vi "ContourExtraction.vi"() -> ()   [LabVIEW 2014]
doc: "This example shows how to use the Edge Tool in NI Vision. The Edge Tool finds edges (or sharp transitions in the pixels values) along a given line or ROI profile. The Edge Tool is a precursor function to many of the gauging and inspection tasks. For example, the location of the edges found along a line profile across an object can interpreted as the boundaries of the object whose dimensions have to be measured for a gauging application or the presence of a crack in the surface of an object for an inspection application."
uses:
  <vilib>/vision/Contour.llb/IMAQ Contour Curve Extraction.ctl
  <vilib>/vision/Contour.llb/IMAQ Connect Range Setting.ctl
  <vilib>/vision/NI_Vision_Development_Module.lvlib
panel:
  in  "Contour Selection":T1(ring)
  in  "Search Direction":T2(ring)
  in  "Curve Connection":T3[](array[typedef])=[{"Match Constraints"=0, "Min"=0.0, "Max"=25.0}, {"Match Constraints"=1, "Min"=0.0, "Max"=180.0}, {"Match Constraints"=2, "Min"=0.0, "Max"=25.0}, {"Match Constraints"=3, "Min"=0.0, "Max"=180.0}] {"Max" format="%.2f"; "Min" format="%.2f"; "Match Constraints" items=["Distance (pixel)", "Angle Difference (degrees)", "Connectivity Distance (pixel)", "Gradient Difference (degrees)"]}
  in  "Curve Extraction":T4={"Extraction Mode"=0, "Edge Threshold"=128, "Edge Filter Size"=2, "Min Length"=25, "Search Step Size"=10, "Max Endpoint Gap"=10, "Subpixel"=TRUE} {"Extraction Mode" items=["Normal", "Uniform Regions"]; "Edge Filter Size" items=["Fine", "Normal", "Contour Tracing"]; "Max Endpoint Gap" min=0; "Search Step Size" min=1 max=255 step=1; "Min Length" min=0; "Edge Threshold" min=1 max=350 step=1}
  out "Image":T5(plugin-control)
  in  "Stop":bool
  # "Range"
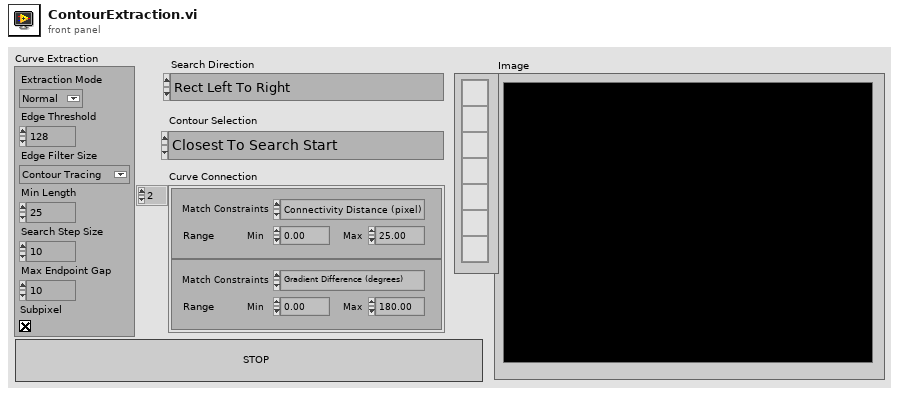
[diagram p1: front panel]
types:
  T1 = enum16{"Closest To Search Start", "Maximum Length", "Strongest Mean Gradient Change"}
  T2 = enum16{"Rect Left To Right", "Rect Right To Left", "Rect Top To Bottom", "Rect Bottom To Top", "Annulus Inner To Outer", "Annulus Outer To Inner", "Annulus Start Angle To End Angle", "Annulus End Angle To Start Angle"}
  T3 = typedef "IMAQ Connect Range Setting.ctl" = cluster{"Match Constraints":u32, "Min":dbl, "Max":dbl}
  T4 = typedef "IMAQ Contour Curve Extraction.ctl" = cluster{"Extraction Mode":u32, "Edge Threshold":i32, "Edge Filter Size":u32, "Min Length":i32, "Search Step Size":i32, "Max Endpoint Gap":i32, "Subpixel":bool}
  T5 = typedef "IMAQ Image.ctl" = refnum<image>
  T6 = typedef "IMAQ Rectangle" = cluster{"Left":i32, "Top":i32, "Right":i32, "Bottom":i32, "Rotation":dbl}
  T7 = typedef "ROI Descriptor" = cluster{"Global Rectangle":i32[], "Contours":cluster{"ID":enum32{"External", "Internal"}, "Type":u32, "Coordinates":i32[]}[]}
  T8 = cluster{"Curve Extraction":T4, "Curve Connection":T3[], "Search Direction":enum16{"Rect Left To Right", "Rect Right To Left", "Rect Top To Bottom", "Rect Bottom To Top", "Annulus Inner To Outer", "Annulus Outer To Inner", "Annulus Start Angle To End Angle", "Annulus End Angle To Start Angle"}, "Contour Selection":enum16{"Closest To Search Start", "Maximum Length", "Strongest Mean Gradient Change"}}
  T9 = cluster{"Overlay?":bool, "Color":u32, "Width":u32, "Maintain Width?":bool}
  T10 = cluster{"Global Rectangle":i32[], "Contours":cluster{"Contour Type":u32, "ROI Type":u32, "Points":i32[]}[]}
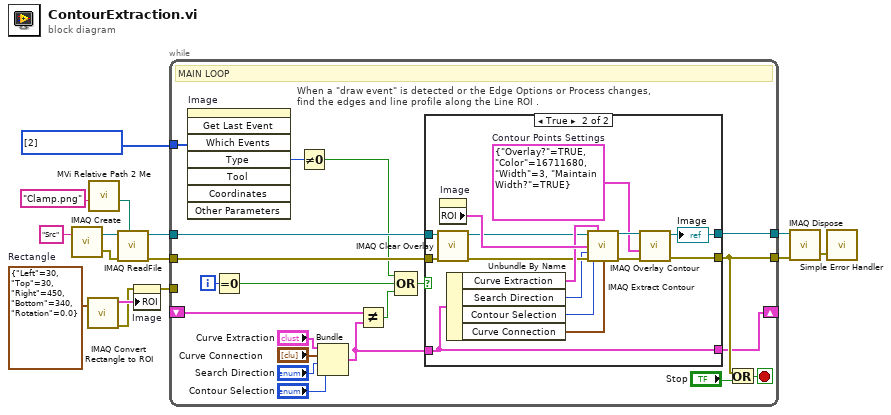
[diagram p0: block diagram]
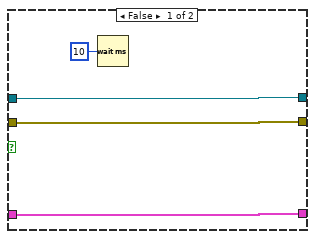
[diagram p2: hidden frame]
diagram:
  w3 = T6 {"Left"=30, "Top"=30, "Right"=450, "Bottom"=340, "Rotation"=0.0}  # Rectangle
  w8 = i32[] [2] items=["No  event", "Click event", "Draw event", "Move event", "Size event", "Scroll event", "Activate event", "Close event", "Double click event"] ("Events list (all)")
  n1 = call "IMAQ Create"("Image Name"="Src") -> ("New Image"=w14:T5, "error out"=w13:errorcluster)  [unwired: 4 in]
  n2 = call "IMAQ Convert Rectangle to ROI"("Rectangle"=w3) -> ("error out"=w2:errorcluster, "ROI Descriptor"=w5:T7)  [unwired: 8 in]
  n3 = call "MVi Relative Path 2 Me.vi"("Relative Path"="Clamp.png" ("name or relative path")) -> ("Appended Dir"=w6:path)  [unwired: 5 in, 1 out]
  n4 = call "IMAQ ReadFile"("File Path"=w6, "error in (no error)"=w13, "Image"=w14) -> ("error out"=w9:errorcluster, "Image Out"=w10:T5)  [unwired: 4 in, 3 out]
  n5 = property on="Image" class="ImageControl"(error in=w2, "ROI"=w5) -> (error out=w4:errorcluster)  [unwired: 1 in, 1 out]
  n6 = while "MAIN LOOP" {
    tunnel: w10 -> [w34]
    tunnel: w9 -> [w35]
    tunnel: [w30] -> w12
    tunnel: [w31] -> w11
    tunnel: w8 -> [w29]
    shift-right: [w24] -> _
    shift-left: _ -> [w21]
    tunnel: w4 -> [_]
    i -> [w27]
    stop <- w32 stop-if-true
    # "When a \"draw event\" is detected or the Edge Options or Process changes, find the edges and line profile along the Line ROI ."
    # "MAIN LOOP"
    n7 = invoke on="Image" class="ImageControl" method="Get Last Event"("Which Events"=w29) -> ("Type"=w28:i32)  [unwired: 7 in, 7 out]
    n8 = Equal To 0?(x=w27) -> (x = 0?=w23:bool)
    n9 = Not Equal To 0?(x=w28) -> (x != 0?=w26:bool)
    n10 = Bundle("Curve Extraction"="Curve Extraction", "Curve Connection"="Curve Connection", "Search Direction"="Search Direction", "Contour Selection"="Contour Selection") -> (w22:T8)  [unwired: 1 in]
    n11 = Not Equal?(x=w21, y=w22) -> (x != y?=w20:bool)
    n12 = Compound Arithmetic op=OR(w26, w23, w20) -> (w25:bool)
    n13 = case shown="True" w25 {
      tunnel: w35 -> [w38 w54]
      tunnel: w34 -> [w39 w53]
      tunnel: [w39 w40] -> w31
      tunnel: [w38 w42] -> w30
      tunnel: [w36 w52] -> w24
      tunnel: w22 -> [w36 w52]
      frame False {
        n14 = Wait (ms)(milliseconds to wait=u32 10) -> ()  [unwired: 1 out]
      }
      frame True {
        w41 = T9 {"Overlay?"=TRUE, "Color"=16711680, "Width"=3, "Maintain Width?"=TRUE}  # Contour Points Settings
        n15 = call "IMAQ Clear Overlay"("error in (no error)"=w54, "Image"=w53) -> ("error out"=w49:errorcluster, "Image Out"=w45:T5)  [unwired: 8 in]
        n16 = property on="Image" class="ImageControl"() -> ("ROI"=w51:T10)  [unwired: 2 in, 2 out]
        n17 = Unbundle By Name(w52) -> ("Curve Extraction"=w50:T4, "Search Direction"=w48:T2, "Contour Selection"=w47:T1, "Curve Connection"=w46:T3[])
        n18 = call "IMAQ Extract Contour"("Source Image"=w45, "Curve Extraction"=w50, "ROI Descriptor"=w51, "Search Direction"=w48, "error in (no error)"=w49, "Contour Selection"=w47, "Curve Connection"=w46) -> ("Source Image Out"=w43:T5, "error out"=w44:errorcluster)  [unwired: 4 in, 3 out]
        n19 = call "IMAQ Overlay Contour"("error in (no error)"=w44, "Contour Points Settings"=w41, "Image"=w43) -> ("error out"=w42:errorcluster, "Image Out"=w40:T5)  [unwired: 3 in, 4 out]
        "Image" <- w40
      }
    }
    n20 = Or(x=w30, y="Stop") -> (x .or. y?=w32:bool)
  }
  n21 = call "IMAQ Dispose"("Image"=w11, "error in (no error)"=w12) -> ("error out"=w1:errorcluster)  [unwired: 4 in]
  n22 = call <vilib>:"Simple Error Handler.vi"("error in (no error)"=w1) -> ()  [unwired: 4 in, 5 out]
